vi "ContMeas - Test.vi"() -> ()   [LabVIEW 2017]
panel:
  out "# elements in queue":i32
  in  "stop":bool
  out "Cont Meas":dbl[](array[numeric])
  out "error out":errorcluster
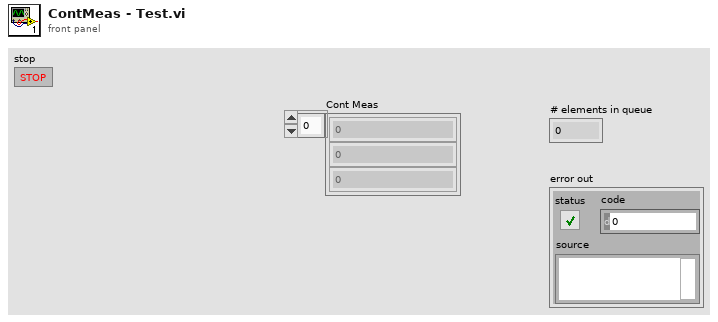
[diagram p1: front panel]
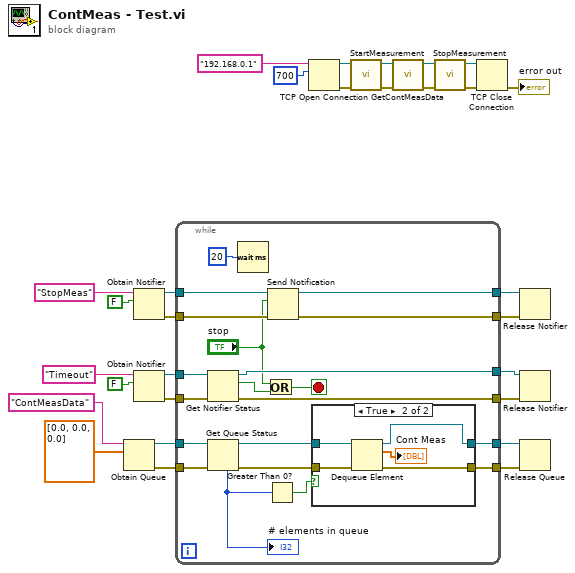
[diagram p0: block diagram]
diagram:
  n1 = Obtain Queue(name (unnamed)="ContMeasData", element data type=dbl[] [0.0, 0.0, 0.0] ("Meas Result")) -> (queue out=w23:refnum<queue>, error out=w22:errorcluster)  [unwired: 3 in, 1 out]
  n2 = Obtain Notifier(name (unnamed)="StopMeas", notification data type=FALSE) -> (notifier out=w18:refnum<notifier>, error out=w17:errorcluster)  [unwired: 2 in, 1 out]
  n3 = Obtain Notifier(name (unnamed)="Timeout", notification data type=FALSE) -> (notifier out=w12:refnum<notifier>, error out=w11:errorcluster)  [unwired: 2 in, 1 out]
  n4 = while {
    tunnel: [w48] -> w24
    tunnel: w23 -> [w47]
    tunnel: w22 -> [w45]
    tunnel: [w49] -> w21
    tunnel: w18 -> [w38]
    tunnel: w17 -> [w37]
    tunnel: [w40] -> w16
    tunnel: [w39] -> w15
    tunnel: w12 -> [w36]
    tunnel: w11 -> [w35]
    tunnel: [w34] -> w10
    tunnel: [w33] -> w9
    stop <- w32 stop-if-true
    n5 = Get Notifier Status(notifier=w36, error in (no error)=w35) -> (notifier out=w34:refnum<notifier>, current notification=w31:bool, error out=w33:errorcluster)  [unwired: 2 out]
    n6 = Get Queue Status(queue=w47, error in (no error)=w45) -> (queue out=w43:refnum<queue>, error out=w44:errorcluster, # elements in queue=w46:i32)  [unwired: 1 in, 5 out]
    "# elements in queue" <- w46
    n7 = Wait (ms)(milliseconds to wait=u32 20) -> ()  [unwired: 1 out]
    n8 = Or(x="stop", y=w31) -> (x .or. y?=w32:bool)
    n9 = Greater Than 0?(x=w46) -> (x > 0?=w42:bool)
    n10 = Send Notification(notification="stop", notifier=w38, error in (no error)=w37) -> (notifier out=w40:refnum<notifier>, error out=w39:errorcluster)
    n11 = case shown="True" w42 {
      tunnel: [w50 w56] -> w49
      tunnel: [w51 w55] -> w48
      tunnel: w44 -> [w50 w52]
      tunnel: w43 -> [w51 w53]
      frame False {
      }
      frame True {
        n12 = Dequeue Element(queue=w53, error in (no error)=w52) -> (queue out=w55:refnum<queue>, element=→"Cont Meas":dbl[], error out=w56:errorcluster)  [unwired: 1 in, 1 out]
      }
    }
  }
  n13 = TCP Open Connection(address="192.168.0.1", remote port or service name=u16 700) -> (connection ID=w4:refnum<k5>, error out=w3:errorcluster)  [unwired: 3 in]
  n14 = call "StartMeasurement.vi"("error in (no error)"=w3, "TCP Network Connection in"=w4) -> ("error out"=w8:errorcluster, "TCP Network Connection out"=w7:refnum<k5>)  [unwired: 6 in, 2 out]
  n15 = call "GetContMeasData.vi"("error in (no error)"=w8, "TCP Network Connection in"=w7) -> ("error out"=w5:errorcluster, "TCP Network Connection out"=w6:refnum<k5>)  [unwired: 6 in, 2 out]
  n16 = call "StopMeasurement.vi"("error in (no error)"=w5, "TCP Network Connection in"=w6) -> ("error out"=w1:errorcluster, "TCP Network Connection out"=w2:refnum<k5>)  [unwired: 6 in, 2 out]
  n17 = TCP Close Connection(connection ID=w2, error in (no error)=w1) -> (error out=→"error out":errorcluster)  [unwired: 1 in, 1 out]
  n18 = Release Notifier(notifier=w16, error in (no error)=w15) -> ()  [unwired: 1 in, 3 out]
  n19 = Release Notifier(notifier=w10, error in (no error)=w9) -> ()  [unwired: 1 in, 3 out]
  n20 = Release Queue(queue=w24, error in (no error)=w21) -> ()  [unwired: 1 in, 3 out]
